vi "Destructor.vi"(8 "error in":errorcluster, 11 "StringMeasure":refnum<class "StringMeasure.lvclass">) -> (0 "error out":errorcluster)   [LabVIEW 2021, in "ProligentXMLGenerator.lvlib" / "StringMeasure.lvclass"]
uses:
  StringMeasure.lvclass
  StringMeasure.lvclass/StringMeasure.ctl
  Measure/Measure.lvclass
  MeasureLimit/MeasureLimit.lvclass
  StringMeasureLimit/StringMeasureLimit.lvclass
  C:/Projects/proligent-xml-generator-labview/src/ProligentXMLGenerator/Measure/Measure/Measure.lvclass
  C:/Projects/proligent-xml-generator-labview/src/ProligentXMLGenerator/Measure/StringMeasure/StringMeasure.lvclass
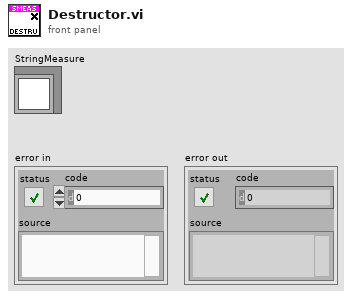
[diagram p1: front panel]
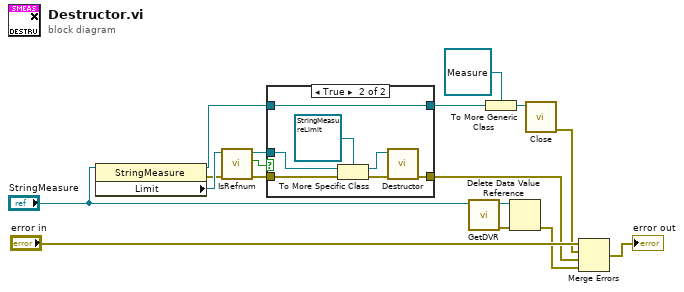
[diagram p0: block diagram]
diagram:
  n1 = property on="Property Node" class="StringMeasure"(reference="StringMeasure") -> (reference out=w5:refnum<class "StringMeasure.lvclass">, error out=w6:errorcluster, "Limit"=w7:refnum<class "MeasureLimit.lvclass">)  [unwired: 1 in]
  n2 = call "IsRefnum.vi"("error in"=w6, "MeasureLimit in"=w7) -> ("error out"=w10:errorcluster, "IsRefnum"=w8:bool, "MeasureLimit out"=w9:refnum<class "MeasureLimit.lvclass">)  [unwired: 7 in]
  n3 = case shown="True" w8 {
    tunnel: w10 -> [w19 w25]
    tunnel: w9 -> [_ w24]
    tunnel: [w19 w22] -> w1
    tunnel: [w18 w26] -> w3
    tunnel: w5 -> [w18 w26]
    frame False {
    }
    frame True {
      n4 = To More Specific Class(target class=refnum<class "StringMeasureLimit.lvclass"> refnum ("ProligentResultProcessor:StringMeasureLimit"), reference=w24, error in=w25) -> (specific class reference=w21:refnum<class "StringMeasureLimit.lvclass">, error out=w23:errorcluster)
      n5 = call "Destructor.vi"("error in"=w23, "StringMeasureLimit"=w21) -> ("error out"=w22:errorcluster)  [unwired: 9 in]
    }
  }
  n6 = call "GetDVR.vi"("StringMeasure"="StringMeasure") -> ("error out"=w14:errorcluster, "DVRReference"=w15:refnum<data-value>)  [unwired: 9 in]
  n7 = To More Generic Class(target class=refnum<class "Measure.lvclass"> refnum ("ProligentResultProcessor:Measure"), reference=w3) -> (generic class reference=w11:refnum<class "Measure.lvclass">)
  n8 = Delete Data Value Reference(data value reference=w15, error in=w14) -> (error out=w12:errorcluster)  [unwired: 1 out]
  n9 = call "Close.vi"("Measure"=w11) -> ("error out"=w13:errorcluster)  [unwired: 10 in]
  n10 = Merge Errors("error in", w13, w1, w12) -> (→"error out":errorcluster)
